vi "Write Motor_Parameters.vi"(8 "error in (no error)":errorcluster, 10 "motor parameters":T1, 11 "Motor in":refnum<class "Motor.lvclass">) -> (0 "error out":errorcluster, 3 "Motor out":refnum<class "Motor.lvclass">)   [LabVIEW 2016, in "Hardware.lvlib" / "Motor.lvlib" / "Motor.lvclass"]
uses:
  <userlib>/Common Components/Hardware/Motor/Motor/Motor.lvclass
  <userlib>/Common Components/Hardware/Motor/Motor/Motor_Parameters.ctl
  <userlib>/Common Components/Hardware/Motor/Motor/Motor.lvclass/Motor.ctl
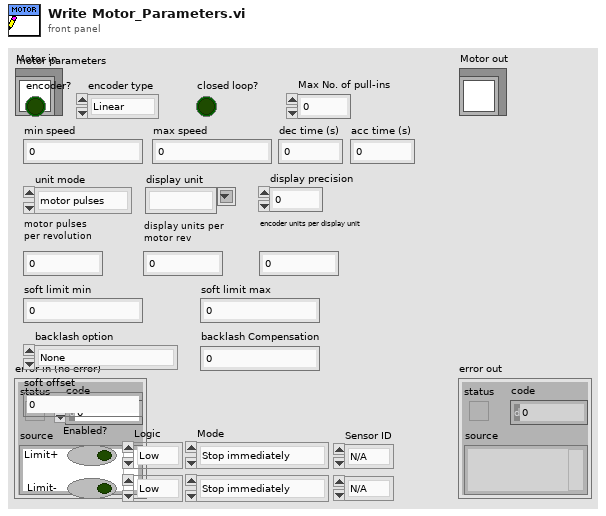
[diagram p1: front panel]
types:
  T1 = typedef "Hardware.lvlib/Motor.lvlib/Motor.lvclass/Motor_Parameters.ctl" = cluster{"closed loop?":bool, "encoder?":bool, "min speed":dbl, "max speed":dbl, "acc time (s)":dbl, "dec time (s)":dbl, "unit mode":enum16{"motor pulses", "real world"}, "motor pulses per revolution":dbl, "display units per motor rev":dbl, "encoder units ratio":dbl, "display unit":string, "display precision":u8, "soft limit min":dbl, "soft limit max":dbl, "Max No. of pull-ins":u8, "Limit+":bool, "Limit+ Logic":enum16{"Low", "High"}, "Limit+ Mode":enum16{"Stop immediately", "Decelerate to Stop"}, "Limit-":bool, "Limit- Logic":enum16{"Low", "High"}, "Limit- Mode":enum16{"Stop immediately", "Decelerate to Stop"}, "Limit+ Sensor ID":enum16{"N/A", "S1", "S2", "S3"}, "Limit- Sensor ID":enum16{"N/A", "S1", "S2", "S3"}, "backlash Compensation":dbl, "soft offset":dbl, "backlash option":enum16{"None", "arriving in + direction", "arriving in - direction"}, "encoder type":enum16{"Linear", "Rotary"}}
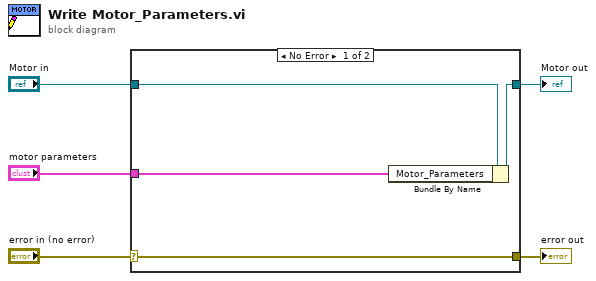
[diagram p0: block diagram]
diagram:
  n1 = case shown="No Error" "error in (no error)" {
    selector: "error in (no error)" -> [w9 w10]
    tunnel: [w9 w10] -> w4
    tunnel: [w7 w11] -> w2
    tunnel: "Motor in" -> [w8 w11]
    tunnel: "motor parameters" -> [w6 _]
    frame No Error {
      n2 = Bundle By Name(cluster=w8, "Motor_Parameters"=w6) -> (w7:refnum<class "Motor.lvclass">)
    }
    frame Error {
    }
  }
  "error out" <- w4
  "Motor out" <- w2
